vi "ma_Hee window.vi"(0 "X":dbl[](array[numeric]) format="%0.2f") -> (1 "Hee {X}":dbl[](array[numeric]) format="%0.2f", 2 "error":i32)   [LabVIEW 2020, in "NI_MAPro.lvlib"]
doc: "Applies a Hanning window to the input sequence X. If Y represents the output sequence, the elements are obtained using the equation\n\n Y[i] = 0.5X[i][1-cos(w)]\n\n where \n w = (2*PI)i/n\n n = the number of elements in X."
uses:
  NI_MAPro.lvlib
  NI_AALPro.lvlib
panel:
  in  "Hee coefficients":dbl[](array[numeric])=[1.0, 1.45875575, 0.54308792, 0.0881675, 0.00390256] format="%0.8f"
  # "Hee Window"
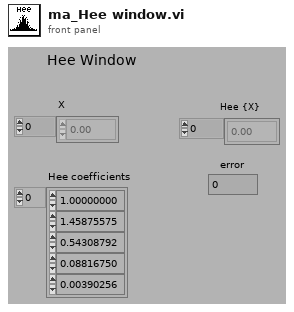
[diagram p1: front panel]
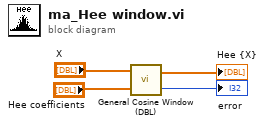
[diagram p0: block diagram]
diagram:
  n1 = call "General Cosine Window (DBL).vi"("Cosine Coefficients"="Hee coefficients", "X"="X") -> ("error"=→"error":i32, "Windowed X"=→"Hee {X}":dbl[])
